vi "Save Current Position to File.vi"(8 "error in (no error)":errorcluster, 9 "file path":path, 10 "Array of axes":T1[](array[typedef]), 11 "VISA in":refnum<visa-resource-name>) -> (0 "error out":errorcluster, 1 "file path out":path, 2 "Array of positions [um]":dbl[](array[numeric]), 3 "VISA out":refnum<visa-resource-name>)   [LabVIEW 2018, in "ASI TG-1000.lvlib"]
doc: "Queries the ASI controller for the position along the specified axes and saves the result to a file for later use."
uses:
  ASI TG-1000.lvlib
  Utility/Axis Name.ctl
  Private/File action if doesn't exist.ctl
  <vilib>/Utility/config.llb/Write Key (Double).vi
  <vilib>/Utility/config.llb/NI_LVConfig.lvlib
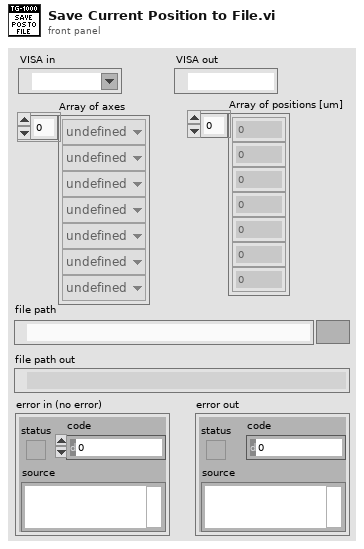
[diagram p1: front panel]
types:
  T1 = typedef "ASI TG-1000.lvlib/Axis Name.ctl" = enum8{"undefined", "A", "B", "C", "D", "E", "F", "G", "H", "I", "J", "K", "L", "M", "N", "O", "P", "Q", "R", "S", "T", "U", "V", "W", "X", "Y", "Z"}
  T2 = typedef "ASI TG-1000.lvlib/File action if doesn't exist.ctl" = enum16{"prompt for existing", "try to create, prompt if can't", "try to create, error if can't"}
  T3 = typedef "NI_LVConfig.lvlib/Config Data RefNum.ctl" = refnum<k1>
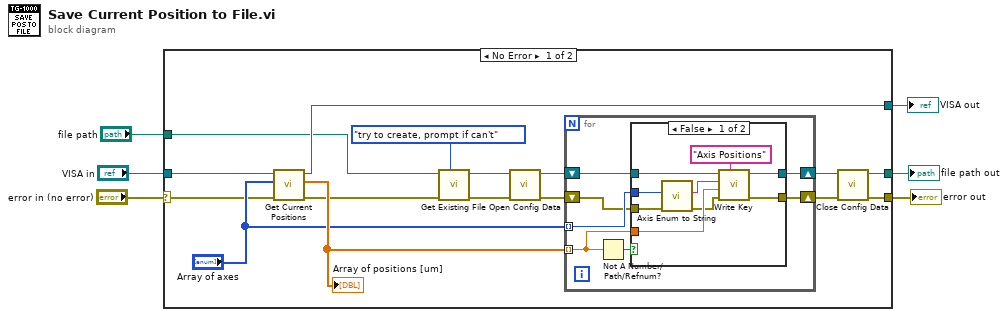
[diagram p0: block diagram]
diagram:
  n1 = case shown="No Error" "error in (no error)" {
    selector: "error in (no error)" -> [w14 w43]
    tunnel: [w18 w43] -> w6
    tunnel: "VISA in" -> [w17 w42]
    tunnel: [w13 w42] -> w3
    tunnel: "file path" -> [w8 w41]
    tunnel: [w7 w41] -> w1
    frame No Error {
      n2 = call "Get Current Positions.vi"("error in (no error)"=w14, "Array of axes"="Array of axes", "VISA in"=w17) -> ("error out"=w12:errorcluster, "Array of positions [internal units]"=w16:dbl[], "VISA out"=w13:refnum<visa-resource-name>)  [unwired: 6 in]
      "Array of positions [um]" <- w16
      n3 = call "Get Existing File.vi"("action if file doesn't exist (0: prompt for existing)"=File_action_if_doesn't_exist."try to create, prompt if can't" ("action if doesn't exist (0: prompt for existing)"), "error in (no error)"=w12, "file path in"=w8) -> ("error out"=w11:errorcluster, "file path out"=w10:path)  [unwired: 7 in]
      n4 = call <vilib>:"Open Config Data.vi"("error in (no error)"=w11, "configuration file path"=w10) -> ("error out"=w21:errorcluster, "refnum"=w22:T3)  [unwired: 7 in, 1 out]
      n5 = for {
        tunnel: "Array of axes" -> [w24] mode=indexing
        tunnel: w16 -> [w26] mode=indexing
        shift-right: [w28] -> w20
        shift-left: w22 -> [w29]
        shift-right: [w27] -> w19
        shift-left: w21 -> [w23]
        n6 = Not A Number/Path/Refnum?(number/path/refnum=w26) -> (NaN/Path/Refnum?=w25:bool)
        n7 = case shown="False" w25 {
          tunnel: w29 -> [w38 w40]
          tunnel: w26 -> [w37 _]
          tunnel: [w35 w40] -> w28
          tunnel: [w34 w39] -> w27
          tunnel: w24 -> [w33 _]
          tunnel: w23 -> [w32 w39]
          frame False {
            n8 = call "Axis Enum to String.vi"("error in (no error)"=w32, "Axis Enum In"=w33) -> ("error out"=w31:errorcluster, "Axis String Out"=w30:string)  [unwired: 8 in]
            n9 = call-poly <vilib>:"Write Key.vi"("section"="Axis Positions", "error in (no error)"=w31, "value"=w37, "key"=w30, "refnum"=w38) -> ("error out"=w34:errorcluster, "refnum out"=w35:T3)  [unwired: 4 in, 1 out]
          }
          frame True {
          }
        }
      }
      n10 = call <vilib>:"Close Config Data.vi"("error in (no error)"=w19, "refnum"=w20) -> ("error out"=w18:errorcluster, "file path"=w7:path)  [unwired: 8 in]
    }
    frame Error {
    }
  }
  "error out" <- w6
  "VISA out" <- w3
  "file path out" <- w1
